vi "Init.vi"(8 "error in (no error)":errorcluster, 11 "Change Temperature in":refnum<class "Change Temperature.lvclass">) -> (0 "error out":errorcluster, 2 "T DVR":refnum<data-value>, 3 "Change Temperature out":refnum<class "Change Temperature.lvclass">)   [LabVIEW 2015, in "Change Temperature.lvclass"]
uses:
  Change Temperature.lvclass
  Change Temperature.lvclass/Change Temperature.ctl
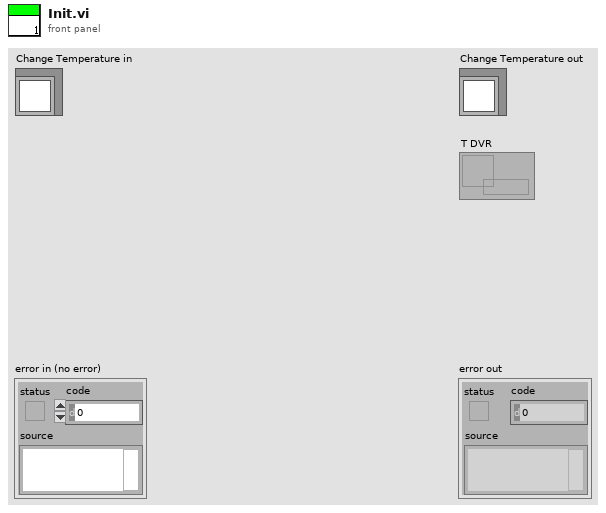
[diagram p1: front panel]
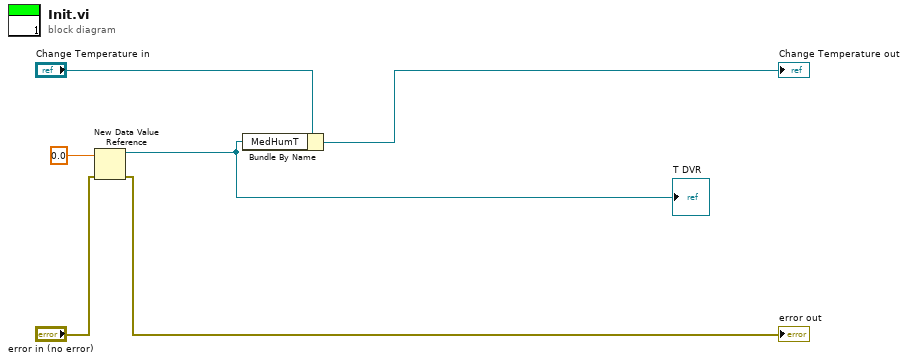
[diagram p0: block diagram]
diagram:
  n1 = New Data Value Reference(data value=0.0, error in="error in (no error)") -> (data value reference=w1:refnum<data-value>, error out=→"error out":errorcluster)
  "T DVR" <- w1
  n2 = Bundle By Name(cluster="Change Temperature in", "MedHumT"=w1) -> (→"Change Temperature out":refnum<class "Change Temperature.lvclass">)
